vi "SaveFile.vi"(10 "data in":u8[](array[numeric]), 11 "File to be opened path":path) -> (3 "opened path":path, 5 "String":string)   [LabVIEW 2016]
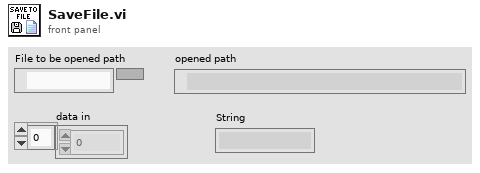
[diagram p1: front panel]
types:
  T1 = enum16{"open", "replace", "create", "open or create", "replace or create", "replace or create with confirmation"}
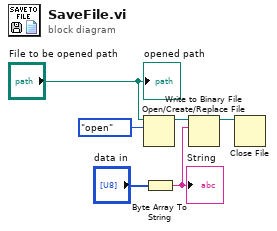
[diagram p0: block diagram]
diagram:
  n1 = Open/Create/Replace File(file path (use dialog)="File to be opened path", operation (0:open)=T1."open") -> (refnum out=w3:refnum<file>)  [unwired: 4 in, 2 out]
  n2 = Byte Array To String(unsigned byte array="data in") -> (string=w1:string)
  "String" <- w1
  n3 = Write to Binary File(file (use dialog)=w3, data=w1) -> (refnum out=w4:refnum<file>)  [unwired: 4 in, 2 out]
  n4 = Close File(refnum=w4) -> ()  [unwired: 1 in, 2 out]
  "opened path" <- "File to be opened path"
